vi "Celsius_to_Fahrenheit.vi"() -> ()   [LabVIEW 2020]
panel:
  in  "deg Celsius":dbl
  out "deg Fahrenheit":dbl
  # "Convert the Celsius to Fahrenheit"
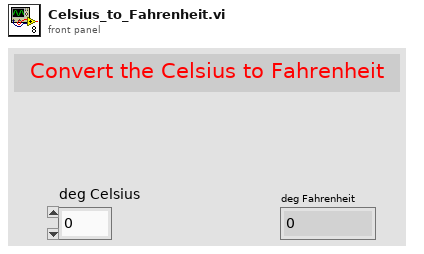
[diagram p1: front panel]
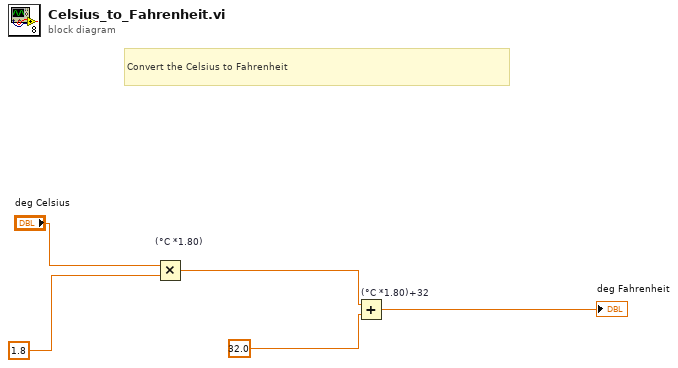
[diagram p0: block diagram]
diagram:
  # "Convert the Celsius to Fahrenheit"
  n1 = Multiply "(°C *1.80)"(x="deg Celsius", y=1.8) -> (x*y=w3:dbl)
  n2 = Add "(°C *1.80)+32"(x=w3, y=32.0) -> (x+y=→"deg Fahrenheit":dbl)
